vi "数据筛选生成condition(子VI).vi"(7 "database data type":T1=enum."Single (SGL)", 8 "Single":cluster{"起始范围":string, "截止范围":string}, 9 "段名":string, 10 "筛选内容":string[](array[string]), 11 "簇转数组":bool[](array[boolean])) -> (3 "condition":string)   [LabVIEW 2016]
uses:
  <vilib>/addons/database/Auxilliary.llb/DB Tools DataTypes.ctl
  <vilib>/addons/database/NI_Database_API.lvlib
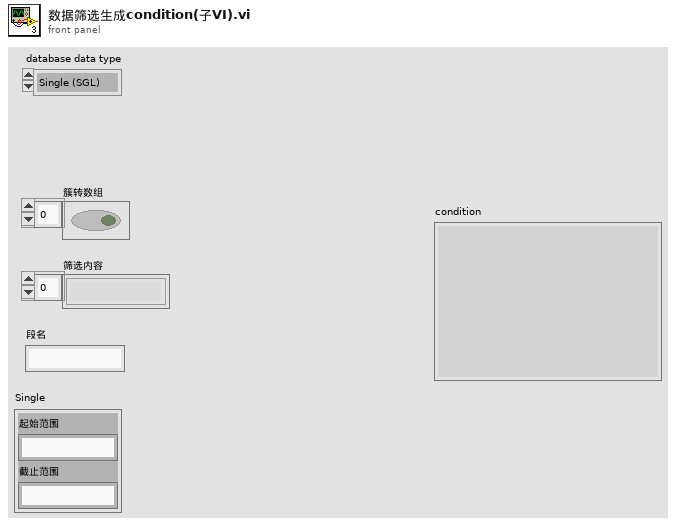
[diagram p1: front panel]
types:
  T1 = typedef "NI_Database_API.lvlib/DB Tools DataTypes.ctl" = enum16{"String", "Long (I32)", "Single (SGL)", "Double (DBL)", "Date/Time", "Binary"}
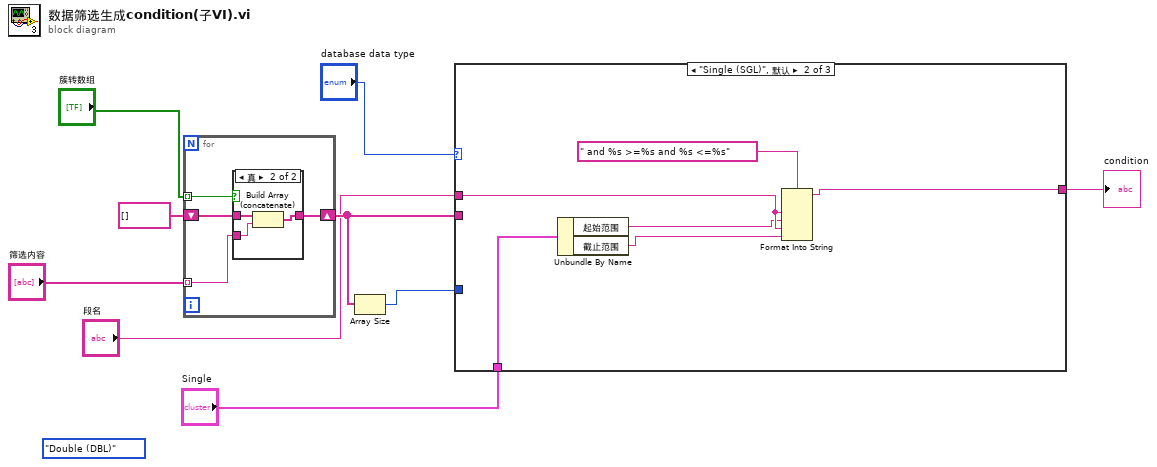
[diagram p0: block diagram]
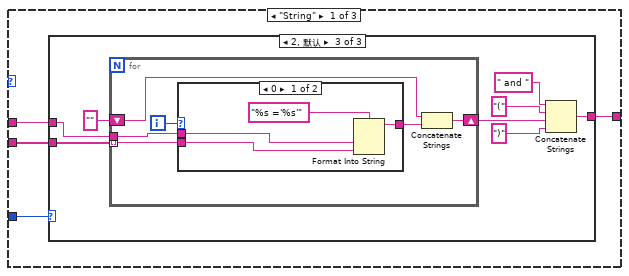
[diagram p2: hidden frame]
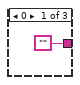
[diagram p3: hidden frame]
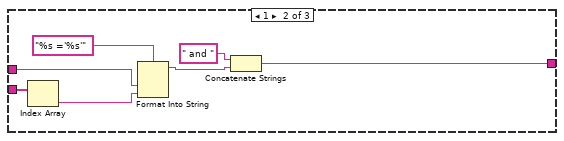
[diagram p4: hidden frame]
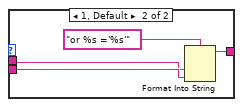
[diagram p5: hidden frame]
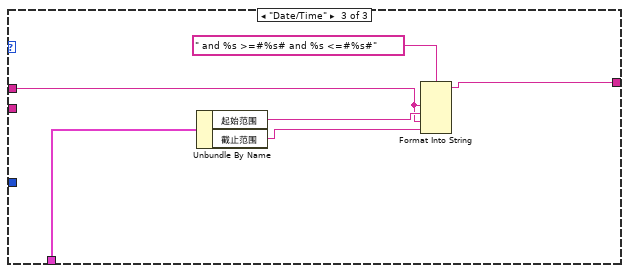
[diagram p6: hidden frame]
diagram:
  (unwired) DB_Tools_DataTypes."Double (DBL)" ("database data type")
  n1 = for {
    tunnel: "簇转数组" -> [w13] mode=indexing
    tunnel: "筛选内容" -> [w12] mode=indexing
    shift-right: [w10] -> w6
    shift-left: string[] [] -> [w11]
    n2 = case shown="真" w13 {
      tunnel: w12 -> [_ w16]
      tunnel: w11 -> [w14 w17]
      tunnel: [w14 w15] -> w10
      frame False {
      }
      frame True {
        n3 = Build Array (concatenate)(w17, w16) -> (w15:string[])
      }
    }
  }
  n4 = Array Size(array=w6) -> (size(s)=w5:i32)
  n5 = case shown="\"Single (SGL)\", 默认" "database data type" {
    tunnel: [w21 w52 w58] -> w9
    tunnel: w6 -> [w20 _ _]
    tunnel: w5 -> [w19 _ _]
    tunnel: "段名" -> [w18 w55 w59]
    tunnel: "Single" -> [_ w57 w60]
    frame "String" {
      n6 = case shown="2, 默认" w19 {
        tunnel: ["" w25 w31] -> w21
        tunnel: w20 -> [_ w27 w37]
        tunnel: w18 -> [_ w23 w30]
        frame 0 {
        }
        frame 1 {
          n7 = Index Array(array=w27) -> (element=w24:string)  [unwired: 1 in]
          n8 = Format Into String(format string="%s ='%s'", w23, w24) -> (resulting string=w26:string)  [unwired: 2 in, 1 out]
          n9 = Concatenate Strings(" and " ("字符串"), w26) -> (w25:string)
        }
        frame 2, Default {
          n10 = for {
            tunnel: w37 -> [w42] mode=indexing
            shift-right: [w41] -> w32
            shift-left: "" -> [w39]
            tunnel: w30 -> [w38]
            i -> [w43]
            n11 = case shown="0" w43 {
              tunnel: w42 -> [w45 w49]
              tunnel: [w46 w50] -> w40
              tunnel: w38 -> [w44 w48]
              frame 0 {
                n12 = Format Into String(format string="%s ='%s'", w44, w45) -> (resulting string=w46:string)  [unwired: 2 in, 1 out]
              }
              frame 1, Default {
                n13 = Format Into String(format string="or %s ='%s'", w48, w49) -> (resulting string=w50:string)  [unwired: 2 in, 1 out]
              }
            }
            n14 = Concatenate Strings(w39, w40) -> (w41:string)
          }
          n15 = Concatenate Strings(" and " ("字符串"), "(" ("字符串"), w32, ")" ("字符串")) -> (w31:string)
        }
      }
    }
    frame "Single (SGL)", Default {
      n16 = Unbundle By Name(w57) -> ("起始范围"=w54:string, "截止范围"=w53:string)
      n17 = Format Into String(format string=" and %s >=%s and %s <=%s", w55, w54, w55, w53) -> (resulting string=w52:string)  [unwired: 2 in, 1 out]
    }
    frame "Date/Time" {
      n18 = Unbundle By Name(w60) -> ("起始范围"=w62:string, "截止范围"=w61:string)
      n19 = Format Into String(format string=" and %s >=#%s# and %s <=#%s#", w59, w62, w59, w61) -> (resulting string=w58:string)  [unwired: 2 in, 1 out]
    }
  }
  "condition" <- w9
